vi "Global_Quit.vi"() -> ()   [LabVIEW 2019]
panel:
  in  "Quit":bool
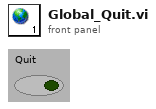
[diagram p1: front panel]
diagram:
